vi "Periodic Tasks.vi"(8 "error in":errorcluster) -> ()   [LabVIEW 2015]
doc: "This VI runs in parallel to other tasks. It can contain as many user-defined periodic loops as you need. These can carry out PID or other sorts of timed response."
uses:
  <vilib>/Rock Robotics/SystemInterfaces/AI/FPGA_AIChannel.ctl
  <vilib>/Rock Robotics/WPI/Utilities/WPI_GetSetVariantRefNum.vi
  <vilib>/Rock Robotics/Network Tables/NT Read Boolean.vi
  <vilib>/Rock Robotics/Network Tables/NT Read Number.vi
  Robot Global Data.vi
  <vilib>/Rock Robotics/Network Tables/NT Write Boolean.vi
  <vilib>/Rock Robotics/Network Tables/NT Write Number.vi
  <vilib>/Rock Robotics/WPI/RobotDrive/WPI_RobotDriveArcadeDrive_Standard(NoSaturation).vi
panel:
  in  "Drive mode":string(combo)="Joystick Control"
  out "Angle":dbl(knob) scale=0.0..360.0
  in  "Reset Angle?":bool
  out "Calibrated?":bool
  out "Distance (in) 2":dbl
  out "Encoder Rate (deg/sec) 2":dbl
  out "Distance (in)":dbl
  out "Encoder Rate (deg/sec)":dbl
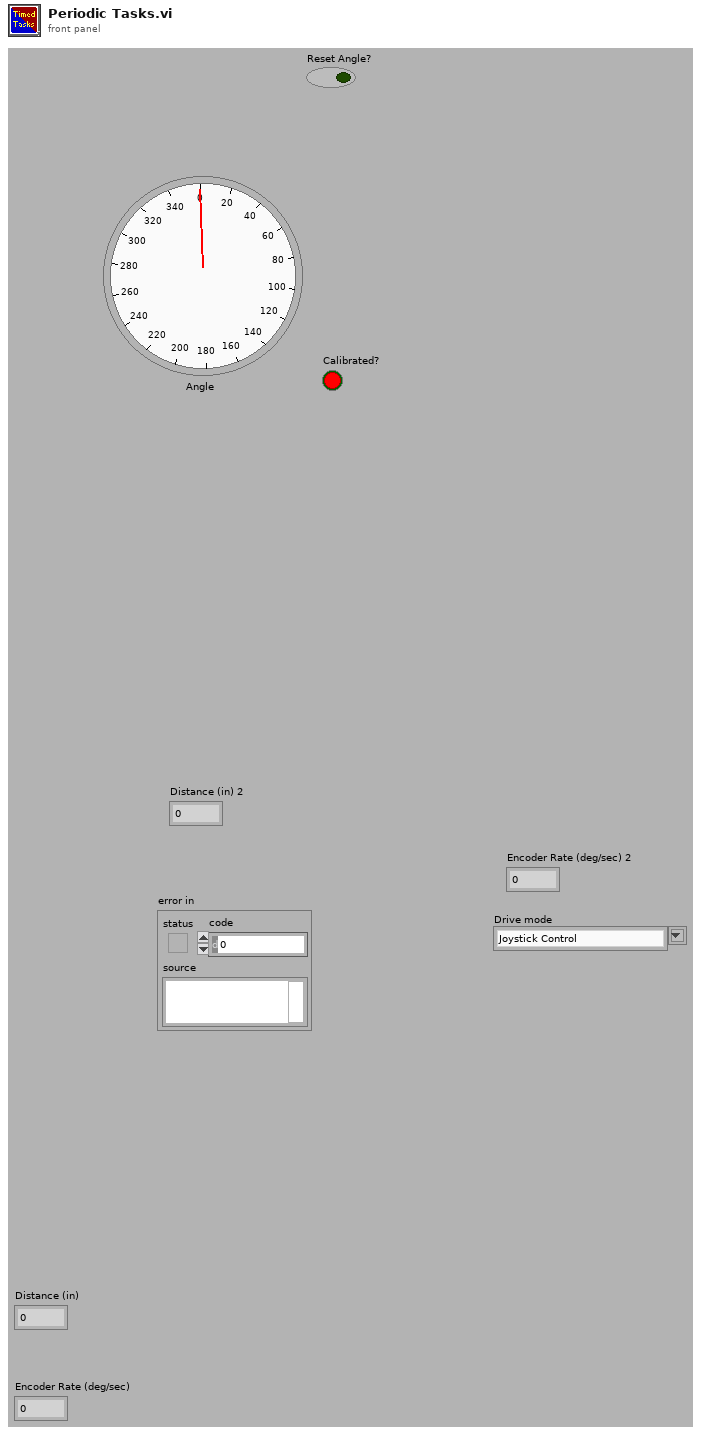
[diagram p1: front panel]
types:
  T1 = typedef "FPGA_AIChannel.ctl" = enum8{"AI 0", "AI 1", "AI 2", "AI 3", "AI MXP 0", "AI MXP 1", "AI MXP 2", "AI MXP 3", "Invalid"}
  T2 = typedef "WPI_MotorControlDeviceRef.ctl" = cluster{"DeviceStatus":errorcluster, "Type":T3, "PWM":cluster{"PWM Channel":T4, "DeadBand":T5}, "CAN":cluster{"Device Number":u8, "Control Mode":T6, "Semaphore":T7, "Max Vout":dbl, "TalonSRX Control Mode":T8}, "Invert":bool}
  T3 = typedef "WPI_MotorControlType.ctl" = enum16{"PWM", "CAN", "CANTalonSRX"}
  T4 = typedef "FPGA_DIOPWMChannel.ctl" = enum8{"PWM 0", "PWM 1", "PWM 2", "PWM 3", "PWM 4", "PWM 5", "PWM 6", "PWM 7", "PWM 8", "PWM 9", "PWM MXP 0", "PWM MXP 1", "PWM MXP 2", "PWM MXP 3", "PWM MXP 4", "PWM MXP 5", "PWM MXP 6", "PWM MXP 7", "PWM MXP 8", "PWM MXP 9", "Invalid"}
  T5 = typedef "WPI_PWMDeadband.ctl" = cluster{"Name":string, "maxPositivePwm":i32, "minPositivePwm":i32, "centerPwm":i32, "maxNegativePwm":i32, "minNegativePwm":i32, "angularRange":u16}
  T6 = typedef "WPI_CANJaguar_ControlMode.ctl" = enum8{"Percent VBus", "Current", "Speed", "Position", "Voltage"}
  T7 = typedef "Semaphore RefNum" = refnum<k1>
  T8 = typedef "WPI_CANTalonSRX_APIControlMode.ctl" = enum8{"Percent VBus", "Speed", "Position", "Slave", "Unchanged / Invalid", "Voltage Compensation", "Current", "Motion Profile"}
  T9 = typedef "WPI_GyroDevRef.ctl" = cluster{"DevStatus":errorcluster, "Analog Channel":T1, "Offset":dbl, "Gain (VoltsPerDegree/Second)":dbl, "Gyro Type":enum16{"Analog", "XRS450"}, "Handle":i32, "SPI Bus":T10, "Device Found":bool, "Sample Rate":dbl, "Calibrate On Open":bool}
  T10 = typedef "spi_bus.ctl" = enum16{"SPI On-Board, CS0", "SPI On-Board, CS1", "SPI On-Board, CS2", "SPI On-Board, CS3", "SPI MXP", "Invalid"}
  T11 = typedef "WPI_JoystickDevRef.ctl" = cluster{"Device":T12}
  T12 = typedef "WPI_JoystickDeviceEnum.ctl" = enum16{"USB 0", "USB 1", "USB 2", "USB 3", "USB 4", "USB 5"}
  T13 = typedef "WPI_RobotDriveDevRef.ctl" = cluster{"DevStatus":errorcluster, "Motors[]":T2[], "Square Inputs":bool, "Max Output":dbl}
  T14 = typedef "WPI_AnalogChannelDevRef.ctl" = cluster{"DevStatus":errorcluster, "Analog Channel":T1}
  T15 = typedef "WPI_EncoderDevRef.ctl" = cluster{"DevStatus":errorcluster, "EncoderIndex":T16, "CounterIndex":T17, "DistancePerCount":dbl, "Decoding Type":T18}
  T16 = typedef "FPGA_EncoderIdx.ctl" = enum8{"Enc 0", "Enc 1", "Enc 2", "Enc 3", "Enc 4", "Enc 5", "Enc 6", "Enc 7", "Invalid"}
  T17 = typedef "FPGA_CounterCtrSystemIndex.ctl" = enum8{"Ctr 0", "Ctr 1", "Ctr 2", "Ctr 3", "Ctr 4", "Ctr 5", "Ctr 6", "Ctr 7", "Invalid"}
  T18 = typedef "WPI_EncoderType.ctl" = enum16{"1x", "2x", "4x"}
  T19 = cluster{"JoystickDevRef":T11, "RobotDriveDevRef":T13}
  T20 = enum16{"Joystick Control", "Drive Straight", "Turn"}
  T21 = enum16{"Roll Ball In", "Stop Roller", "Shoot Ball"}
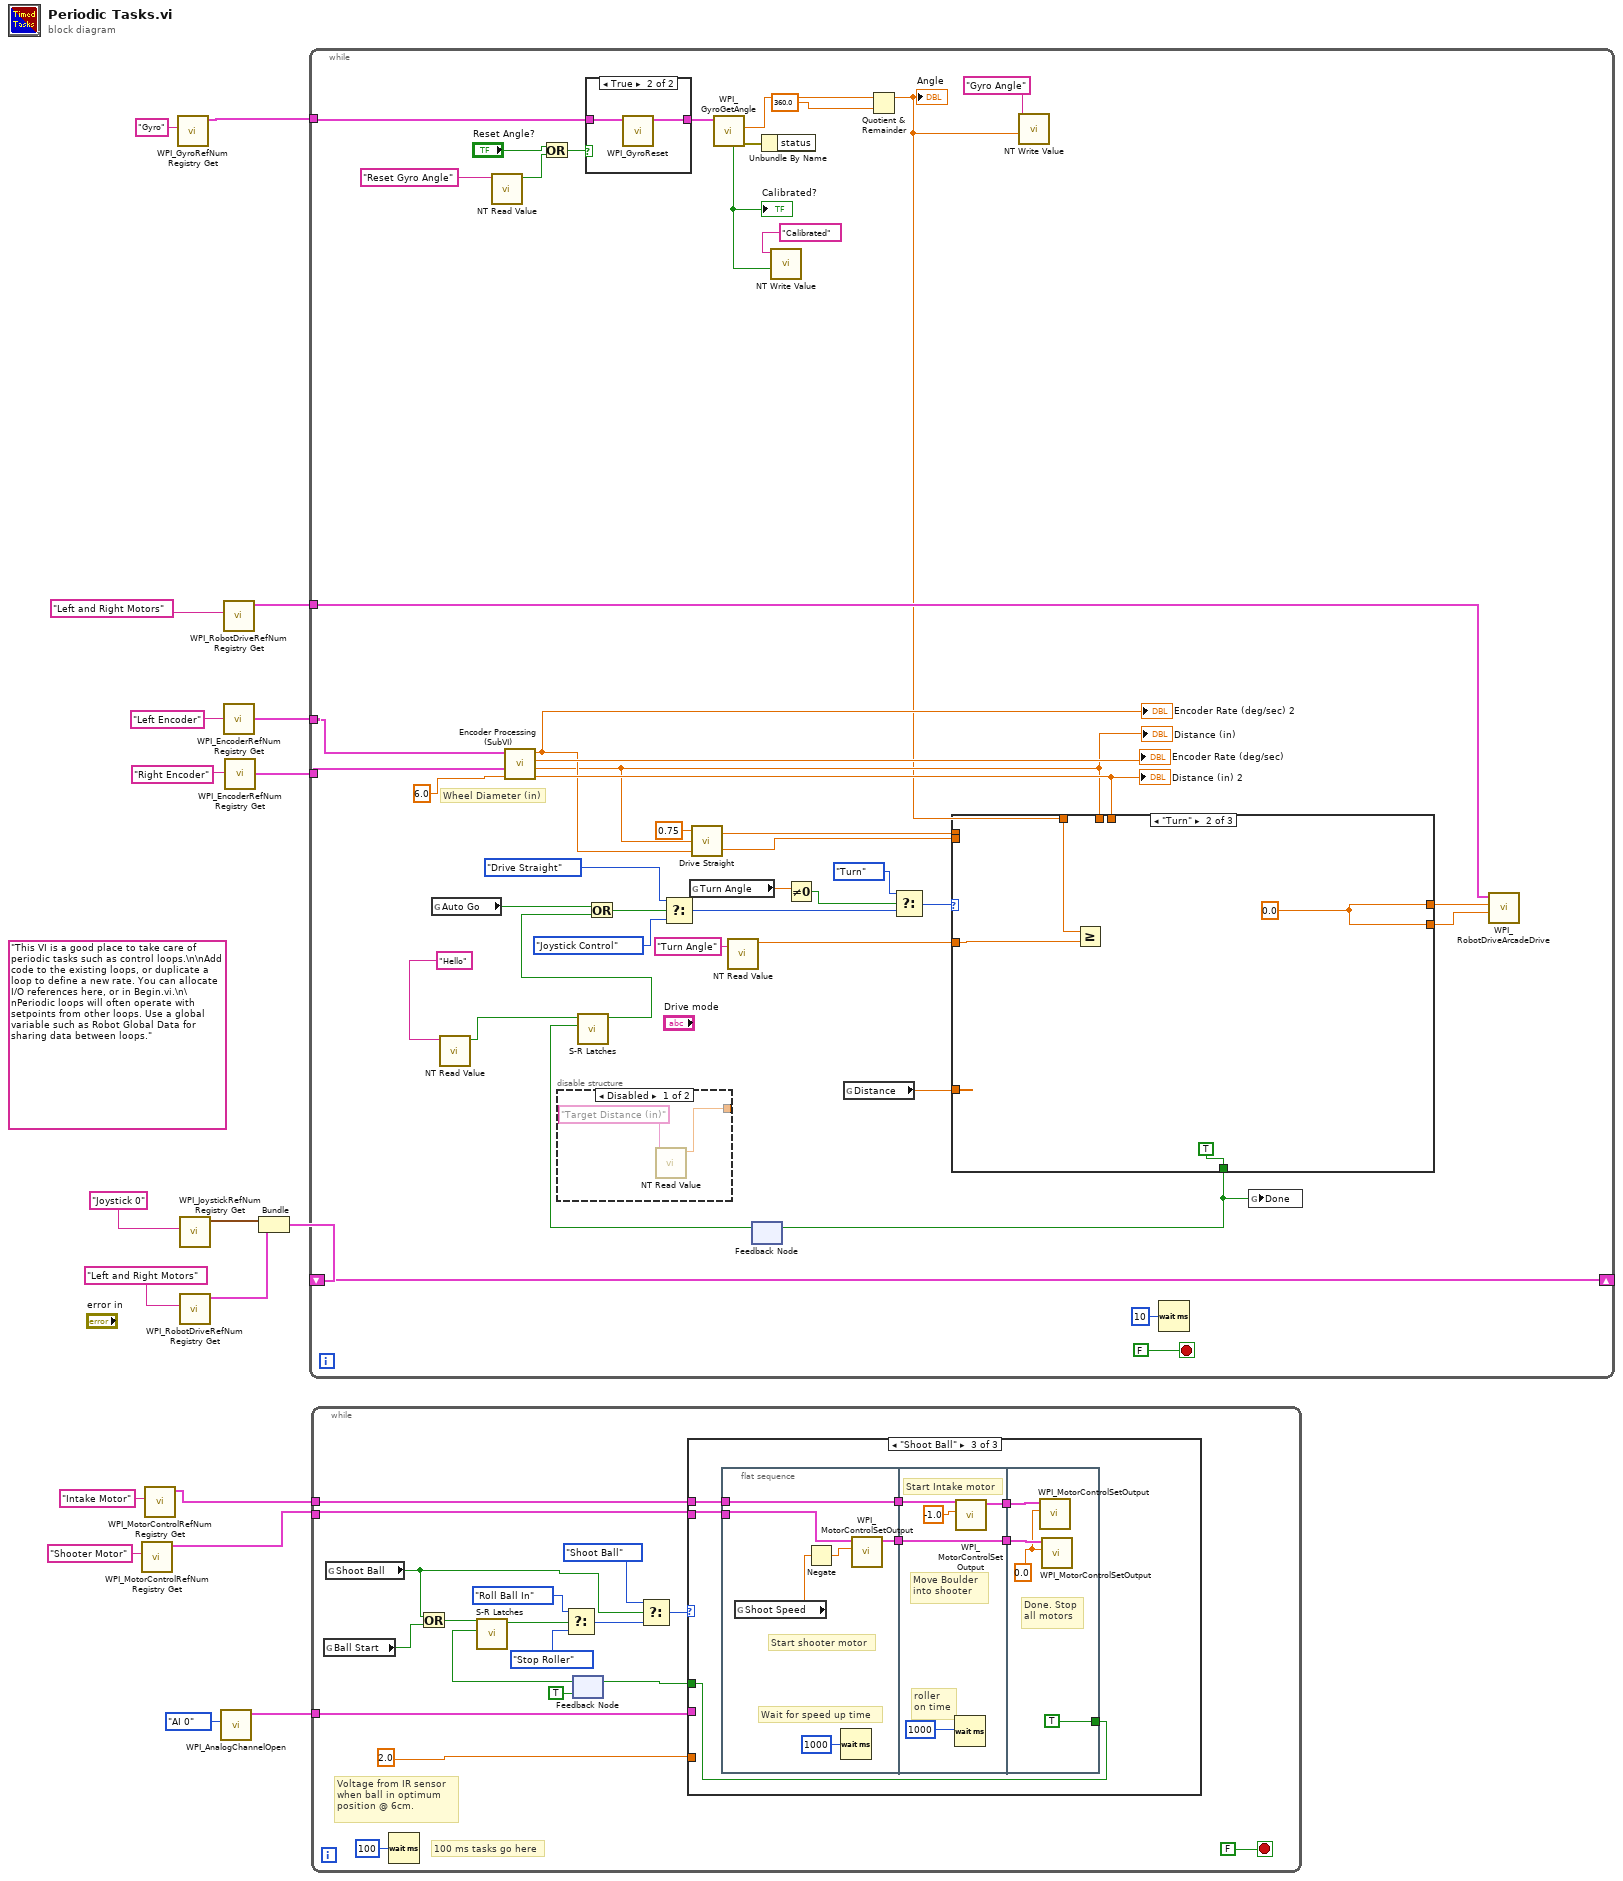
[diagram p0: block diagram]
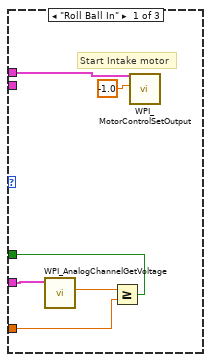
[diagram p2: hidden frame]
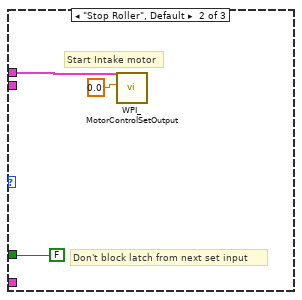
[diagram p3: hidden frame]
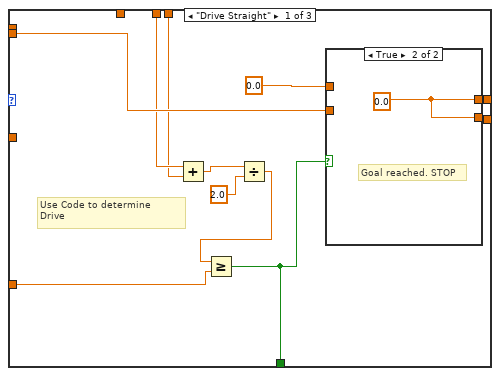
[diagram p5: hidden frame]
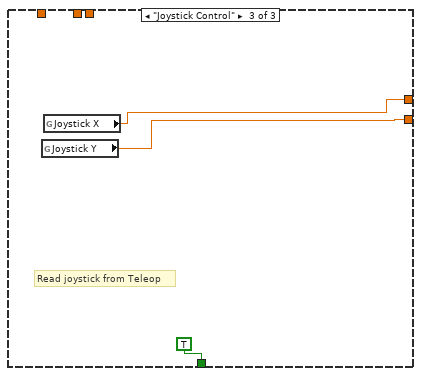
[diagram p7: hidden frame]
diagram:
  (unwired) "This VI is a good place to take care of periodic tasks such as control loops.\n\nAdd code to the existing loops, or duplicate a loop to define a new rate. You can allocate I/O references here, or in Begin.vi.\n\nPeriodic loops will often operate with setpoints from other loops. Use a global variable such as Robot Global Data for sharing data between loops."
  n1 = call <vilib>:"WPI_MotorControlRefNum Registry Get.vi"("refnum name"="Shooter Motor") -> ("MotorControlDevRef"=w6:T2)  [unwired: 9 in, 1 out]
  n2 = call <vilib>:"WPI_MotorControlRefNum Registry Get.vi"("refnum name"="Intake Motor") -> ("MotorControlDevRef"=w5:T2)  [unwired: 9 in, 1 out]
  n3 = call <vilib>:"WPI_GyroRefNum Registry Get.vi"("refnum name"="Gyro") -> ("GyroDevRef"=w8:T9)  [unwired: 9 in, 1 out]
  n4 = call <vilib>:"WPI_JoystickRefNum Registry Get.vi"("refnum name"="Joystick 0") -> ("JoystickDevRef"=w17:T11)  [unwired: 1 in, 9 out]
  n5 = call <vilib>:"WPI_RobotDriveRefNum Registry Get.vi"("refnum name"="Left and Right Motors") -> ("RobotDriveDevRef"=w16:T13)  [unwired: 1 in, 9 out]
  n6 = call <vilib>:"WPI_AnalogChannelOpen.vi"("Analog Channel"=FPGA_AIChannel."AI 0") -> ("AIDeviceRef"=w2:T14)  [unwired: 9 in, 1 out]
  n7 = call <vilib>:"WPI_RobotDriveRefNum Registry Get.vi"("refnum name"="Left and Right Motors") -> ("RobotDriveDevRef"=w9:T13)  [unwired: 9 in, 1 out]
  n8 = call <vilib>:"WPI_EncoderRefNum Registry Get.vi"("refnum name"="Left Encoder") -> ("EncoderDevRef"=w12:T15)  [unwired: 9 in, 1 out]
  n9 = call <vilib>:"WPI_EncoderRefNum Registry Get.vi"("refnum name"="Right Encoder") -> ("EncoderDevRef"=w11:T15)  [unwired: 9 in, 1 out]
  n10 = Bundle("JoystickDevRef"=w17, "RobotDriveDevRef"=w16) -> (w15:T19)  [unwired: 1 out]
  n11 = while {
    shift-right: [w63] -> _
    shift-left: w15 -> [w63]
    tunnel: w12 -> [w62]
    tunnel: w11 -> [w61]
    tunnel: w9 -> [w40]
    tunnel: w8 -> [w60]
    stop <- FALSE stop-if-true
    # "Wheel Diameter (in)"
    n12 = global read "Robot Global Data.vi" "Auto Go"() -> (w26:bool)
    n13 = call-poly <vilib>:"NT Read Value.vi"("Name"="Hello") -> ("Boolean"=w44:bool)  [unwired: 9 in, 1 out]
    n14 = call-poly <vilib>:"NT Read Value.vi"("Name"="Reset Gyro Angle") -> ("Boolean"=w53:bool)  [unwired: 9 in, 1 out]
    n15 = call "Encoder Processing (SubVI).vi"("Wheel Diameter"=6.0, "EncoderDevRef"=w61, "EncoderDevRef 2"=w62) -> ("Distance (in) 2"=w47:dbl, "Distance (in)"=w41:dbl, "Encoder Rate R (deg/sec)"=→"Encoder Rate (deg/sec)":dbl, "Encoder Rate  L(deg/sec) 2"=w42:dbl)  [unwired: 1 in]
    "Distance (in)" <- w41
    "Encoder Rate (deg/sec) 2" <- w42
    "Distance (in) 2" <- w47
    n16 = Or(x="Reset Angle?", y=w53) -> (x .or. y?=w55:bool)
    n17 = disable-structure shown="Disabled" {
      disable-tunnel: [w66 _] -> _
      frame Disabled {
        n18 = call-poly <vilib>:"NT Read Value.vi"("Name"="Target Distance (in)") -> ("Numeric"=w66:dbl)  [unwired: 9 in, 1 out]
      }
      frame Enabled {
      }
    }
    n19 = case shown="True" w55 {
      tunnel: w60 -> [w89 w91]
      tunnel: [w89 w90] -> w58
      frame False {
      }
      frame True {
        n20 = call <vilib>:"WPI_GyroReset.vi"("GyroDevRef"=w91) -> ("GyroDevRef"=w90:T9)  [unwired: 9 in, 1 out]
      }
    }
    n21 = global read "Robot Global Data.vi" "Turn Angle"() -> (w21:dbl)
    n22 = call "Drive Straight.vi"("Rate L"=w42, "Rate R"=w41, "Speed"=0.75) -> ("Y Out"=w48:dbl, "X Out"=w49:dbl)
    n23 = call <vilib>:"WPI_GyroGetAngle.vi"("GyroDevRef"=w58) -> ("error out"=w56:errorcluster, "Angle"=w57:dbl, "Calibrated?"=w35:bool)  [unwired: 6 in, 2 out]
    "Calibrated?" <- w35
    n24 = call-poly <vilib>:"NT Read Value.vi"("Name"="Turn Angle") -> ("Numeric"=w28:dbl)  [unwired: 9 in, 1 out]
    n25 = feedback #1() -> (w37:bool)  [unwired: 1 in]
    n26 = call "S-R Latches.vi"("R1"=w37, "S1"=w44) -> ("Q1"=w30:bool)  [unwired: 4 in, 1 out]
    n27 = Or(x=w26, y=w30) -> (x .or. y?=w34:bool)
    n28 = Select(t=T20."Drive Straight", s=w34, f=T20."Joystick Control") -> (s? t:f=w33:T20)
    n29 = Unbundle By Name(w56) -> ()  [unwired: 1 out]
    n30 = call-poly <vilib>:"NT Write Value.vi"("Boolean"=w35, "Name"="Calibrated") -> ()  [unwired: 9 in, 1 out]
    n31 = Not Equal To 0?(x=w21) -> (x != 0?=w20:bool)
    n32 = global read "Robot Global Data.vi" "Distance"() -> (w25:dbl)
    n33 = Quotient & Remainder(x=w57, y=360.0) -> (x-y*floor(x/y)=w27:dbl)  [unwired: 1 out]
    "Angle" <- w27
    n34 = Select(t=T20."Turn", s=w20, f=w33) -> (s? t:f=w24:T20)
    n35 = case shown="\"Turn\"" w24 {
      tunnel: w49 -> [_ _ _]
      tunnel: w48 -> [w78 _ _]
      tunnel: w41 -> [w77 _ _]
      tunnel: w47 -> [w76 _ _]
      tunnel: [w72 TRUE TRUE] -> w22
      tunnel: [w71 w85 w87] -> w39
      tunnel: [w70 w85 w86] -> w38
      tunnel: w25 -> [w69 _ _]
      tunnel: w28 -> [_ w83 _]
      tunnel: w27 -> [_ w82 _]
      frame "Drive Straight" {
        # "Use Code to determine\nDrive"
        n36 = Add(x=w77, y=w76) -> (x+y=w75:dbl)
        n37 = Divide(x=w75, y=2.0) -> (x/y=w73:dbl)
        n38 = Greater Or Equal?(x=w73, y=w69) -> (x >= y?=w72:bool)
        n39 = case shown="True" w72 {
          tunnel: 0.0 ("X Out") -> [w80 _]
          tunnel: w78 -> [w79 _]
          tunnel: [w80 w81] -> w71
          tunnel: [w79 w81] -> w70
          frame False {
            # "Drive to Goal"
          }
          frame True {
            w81 = 0.0 ("X axis value")
            # "Goal reached. STOP"
          }
        }
      }
      frame "Turn" {
        w85 = 0.0 ("Joystick X")
        n40 = Greater Or Equal?(x=w82, y=w83) -> ()  [unwired: 1 out]
      }
      frame "Joystick Control" {
        # "Read joystick from Teleop"
        n41 = global read "Robot Global Data.vi" "Joystick Y"() -> (w86:dbl)
        n42 = global read "Robot Global Data.vi" "Joystick X"() -> (w87:dbl)
      }
    }
    n43 = feedback-in #1(w22) -> ()
    n44 = call-poly <vilib>:"NT Write Value.vi"("Numeric"=w27, "Name"="Gyro Angle") -> ()  [unwired: 9 in, 1 out]
    n45 = Wait (ms)(milliseconds to wait=u32 10) -> ()  [unwired: 1 out]
    n46 = global write "Robot Global Data.vi" "Done"(w22) -> ()
    n47 = call-poly <vilib>:"WPI_RobotDriveArcadeDrive.vi"("Y axis value"=w38, "X axis value"=w39, "RobotDriveDevRef"=w40) -> ()  [unwired: 6 in, 3 out]
  }
  n48 = while {
    tunnel: w2 -> [w107]
    tunnel: w5 -> [w94]
    tunnel: w6 -> [w93]
    stop <- FALSE stop-if-true
    # "Voltage from IR sensor\nwhen ball in optimum \nposition @ 6cm."
    # "100 ms tasks go here"
    n49 = global read "Robot Global Data.vi" "Ball Start"() -> (w97:bool)
    n50 = global read "Robot Global Data.vi" "Shoot Ball"() -> (w96:bool)
    n51 = Wait (ms)(milliseconds to wait=u32 100) -> ()  [unwired: 1 out]
    n52 = Or(x=w96, y=w97) -> (x .or. y?=w95:bool)
    n53 = feedback #2(TRUE) -> (w102:bool)
    n54 = call "S-R Latches.vi"("R1"=w102, "S1"=w95) -> ("Q1"=w106:bool)  [unwired: 4 in, 1 out]
    n55 = Select(t=T21."Roll Ball In", s=w106, f=T21."Stop Roller") -> (s? t:f=w99:T21)
    n56 = Select(t=T21."Shoot Ball", s=w96, f=w99) -> (s? t:f=w100:T21)
    n57 = case shown="\"Shoot Ball\"" w100 {
      tunnel: w107 -> [w114 _ _]
      tunnel: 2.0 ("Ball Voltage") -> [w113 _ _]
      tunnel: [w112 FALSE w125] -> w103
      tunnel: w94 -> [w110 w116 w124]
      tunnel: w93 -> [_ _ w123]
      frame "Roll Ball In" {
        # "Start Intake motor"
        n58 = call <vilib>:"WPI_AnalogChannelGetVoltage.vi"("AIDeviceRef"=w114) -> ("Voltage"=w115:dbl)  [unwired: 8 in, 2 out]
        n59 = Greater Or Equal?(x=w115, y=w113) -> (x >= y?=w112:bool)
        n60 = call <vilib>:"WPI_MotorControlSetOutput.vi"("Output"=-1.0, "MotorControlDevRef"=w110) -> ()  [unwired: 7 in, 3 out]
      }
      frame "Stop Roller", Default {
        # "Don't block latch from next set input"
        # "Start Intake motor"
        n61 = call <vilib>:"WPI_MotorControlSetOutput.vi"("Output"=0.0, "MotorControlDevRef"=w116) -> ()  [unwired: 7 in, 3 out]
      }
      frame "Shoot Ball" {
        n62 = flat-sequence {
          tunnel: [w128] -> w122
          tunnel: [w129] -> w121
          tunnel: w124 -> [w128]
          tunnel: w123 -> [w127]
          tunnel: w122 -> [w136]
          tunnel: [w134] -> w120
          tunnel: [w133] -> w119
          tunnel: w121 -> [w133]
          tunnel: w120 -> [w140]
          tunnel: w119 -> [w139]
          tunnel: [TRUE] -> w125
          frame #0 {
            # "Wait for speed up time"
            # "Start shooter motor"
            n63 = global read "Robot Global Data.vi" "Shoot Speed"() -> (w131:dbl)
            n64 = Negate(x=w131) -> (-x=w130:dbl)
            n65 = Wait (ms)(milliseconds to wait=u32 1000) -> ()  [unwired: 1 out]
            n66 = call <vilib>:"WPI_MotorControlSetOutput.vi"("Output"=w130, "MotorControlDevRef"=w127) -> ("MotorControlDevRef"=w129:T2)  [unwired: 7 in, 2 out]
          }
          frame #1 {
            # "Move Boulder\ninto shooter"
            # "roller \non time"
            # "Start Intake motor"
            n67 = Wait (ms)(milliseconds to wait=u32 1000 ("y")) -> ()  [unwired: 1 out]
            n68 = call <vilib>:"WPI_MotorControlSetOutput.vi"("Output"=-1.0, "MotorControlDevRef"=w136) -> ("MotorControlDevRef"=w134:T2)  [unwired: 7 in, 2 out]
          }
          frame #2 {
            w138 = 0.0 ("Output")
            # "Done. Stop\nall motors"
            n69 = call <vilib>:"WPI_MotorControlSetOutput.vi"("Output"=w138, "MotorControlDevRef"=w140) -> ()  [unwired: 7 in, 3 out]
            n70 = call <vilib>:"WPI_MotorControlSetOutput.vi"("Output"=w138, "MotorControlDevRef"=w139) -> ()  [unwired: 7 in, 3 out]
          }
        }
      }
    }
    n71 = feedback-in #2(w103) -> ()
  }
